vi "Halvorsen_HDiagram_BasicMethods.vi"(11 "Initial Conditions":ext[](array[numeric])=[0.1, 0.1, 0.1]) -> ()   [LabVIEW 2016]
panel:
  out "Current h":ext=0.9999999999999999994
  in  "Inc h, с":ext=0.01
  in  "Parameters":ext[](array[numeric])=[0.1, 0.0, 0.1]
  in  "Tab Control":enum32{"Mode Analysis", "Time Domain"}(tab)=enum."Time Domain"
  out "Mode Analysis":cluster{ext[], dbl[]}[](graph)=[{[0.01, 0.02, 0.03, 0.04, 0.049999999999999999997, 0.059999999999999999995, 0.069999999999999999993, 0.07999999999999999999, 0.08999999999999999999, 0.09999999999999999999, 0.109999999999999999986, 0.119999999999999999984, 0.12999999999999999998, 0.13999999999999999999, 0.14999999999999999999, 0.16, 0.17, 0.18000000000000000001, 0.19000000000000000001, 0.20000000000000000002, 0.21000000000000000002, 0.22000000000000000003, 0.23000000000000000003, 0.24000000000000000004, 0.25000000000000000003, 0.26000000000000000002, 0.27000000000000000001, 0.28, 0.29, 0.29999999999999999998, 0.30999999999999999998, 0.31999999999999999997, 0.32999999999999999996, 0.33999999999999999995, 0.34999999999999999994, 0.35999999999999999993, 0.36999999999999999992, 0.37999999999999999991, 0.3899999999999999999, 0.3999999999999999999, 0.40999999999999999989, 0.41999999999999999988, 0.42999999999999999987, 0.43999999999999999986, 0.44999999999999999985, 0.45999999999999999984, 0.46999999999999999984, 0.47999999999999999983, 0.48999999999999999982, 0.4999999999999999998, 0.50999999999999999983, 0.51999999999999999982, 0.5299999999999999998, 0.5399999999999999998, 0.5499999999999999998, 0.5599999999999999998, 0.56999999999999999978, 0.57999999999999999977, 0.58999999999999999976, 0.59999999999999999975, 0.60999999999999999974, 0.61999999999999999973, 0.62999999999999999972, 0.6399999999999999997, 0.6499999999999999997, 0.6599999999999999997, 0.6699999999999999997, 0.67999999999999999968, 0.68999999999999999967, 0.69999999999999999966, 0.70999999999999999966, 0.71999999999999999965, 0.72999999999999999964, 0.73999999999999999963, 0.74999999999999999962, 0.7599999999999999996, 0.7699999999999999996, 0.7799999999999999996, 0.7899999999999999996, 0.79999999999999999958, 0.80999999999999999957, 0.81999999999999999956, 0.82999999999999999955, 0.83999999999999999954, 0.84999999999999999953, 0.85999999999999999953, 0.8699999999999999995, 0.8799999999999999995, 0.8899999999999999995, 0.8999999999999999995, 0.9099999999999999995, 0.91999999999999999947, 0.92999999999999999946, 0.93999999999999999946, 0.94999999999999999945, 0.95999999999999999944, 0.96999999999999999943, 0.9799999999999999994, 0.9899999999999999994], [1.0, 1.0, 1.0, 1.0, 1.0, 1.0, 1.0, 1.0, 1.0, 1.0, 1.0, 1.0, 1.0, 1.0, 1.0, 1.0, 1.0, 1.0, 1.0, 1.0, 1.0, 1.0, 1.0, 1.0, 1.0, 1.0, 1.0, 1.0, 1.0, 1.0, 1.0, 1.0, 1.0, 1.0, 1.0, 1.0, 1.0, 1.0, 1.0, 1.0, 1.0, 1.0, 1.0, 1.0, 1.0, 1.0, 1.0, 1.0, 1.0, 1.0, 1.0, 1.0, 1.0, 1.0, 1.0, 1.0, 1.0, 1.0, 1.0, 1.0, 1.0, 1.0, 1.0, 1.0, 1.0, 1.0, 1.0, 1.0, 1.0, 1.0, 1.0, 22.0, 1.0, 1.0, 1.0, 1.0, 1.0, 18.0, 1.0, 1.0, 1.0, 1.0, 1.0, 1.0, 1.0, 1.0, 1.0, 24.0, 1.0, 1.0, 1.0, 1.0, 1.0, 1.0, 1.0, 1.0, 1.0, 1.0, 1.0]}, {[0.01, 0.02, 0.03, 0.04, 0.049999999999999999997, 0.059999999999999999995, 0.069999999999999999993, 0.07999999999999999999, 0.08999999999999999999, 0.09999999999999999999, 0.109999999999999999986, 0.119999999999999999984, 0.12999999999999999998, 0.13999999999999999999, 0.14999999999999999999, 0.16, 0.17, 0.18000000000000000001, 0.19000000000000000001, 0.20000000000000000002, 0.21000000000000000002, 0.22000000000000000003, 0.23000000000000000003, 0.24000000000000000004, 0.25000000000000000003, 0.26000000000000000002, 0.27000000000000000001, 0.28, 0.29, 0.29999999999999999998, 0.30999999999999999998, 0.31999999999999999997, 0.32999999999999999996, 0.33999999999999999995, 0.34999999999999999994, 0.35999999999999999993, 0.36999999999999999992, 0.37999999999999999991, 0.3899999999999999999, 0.3999999999999999999, 0.40999999999999999989, 0.41999999999999999988, 0.42999999999999999987, 0.43999999999999999986, 0.44999999999999999985, 0.45999999999999999984, 0.46999999999999999984, 0.47999999999999999983, 0.48999999999999999982, 0.4999999999999999998, 0.50999999999999999983, 0.51999999999999999982, 0.5299999999999999998, 0.5399999999999999998, 0.5499999999999999998, 0.5599999999999999998, 0.56999999999999999978, 0.57999999999999999977, 0.58999999999999999976, 0.59999999999999999975, 0.60999999999999999974, 0.61999999999999999973, 0.62999999999999999972, 0.6399999999999999997, 0.6499999999999999997, 0.6599999999999999997, 0.6699999999999999997, 0.67999999999999999968, 0.68999999999999999967, 0.69999999999999999966, 0.70999999999999999966, 0.71999999999999999965, 0.72999999999999999964, 0.73999999999999999963, 0.74999999999999999962, 0.7599999999999999996, 0.7699999999999999996, 0.7799999999999999996, 0.7899999999999999996, 0.79999999999999999958, 0.80999999999999999957, 0.81999999999999999956, 0.82999999999999999955, 0.83999999999999999954, 0.84999999999999999953, 0.85999999999999999953, 0.8699999999999999995, 0.8799999999999999995, 0.8899999999999999995, 0.8999999999999999995, 0.9099999999999999995, 0.91999999999999999947, 0.92999999999999999946, 0.93999999999999999946, 0.94999999999999999945, 0.95999999999999999944, 0.96999999999999999943, 0.9799999999999999994, 0.9899999999999999994], [0.0, 0.0, 0.0, 0.0, 0.0, 0.0, 0.0, 0.0, 0.0, 0.0, 0.0, 0.0, 0.0, 0.0, 0.0, 0.0, 0.0, 0.0, 0.0, 0.0, 0.0, 0.0, 0.0, 0.0, 0.0, 0.0, 0.0, 0.0, 0.0, 0.0, 0.0, 0.0, 0.0, 0.0, 0.0, 0.0, 0.0, 0.0, 0.0, 0.0, 0.0, 0.0, 0.0, 0.0, 0.0, 0.0, 0.0, 0.0, 0.0, 0.0, 0.0, 0.0, 0.0, 0.0, 0.0, 0.0, 0.0, 0.0, 0.0, 0.0, 0.0, 0.0, 0.0, 0.0, 0.0, 0.0, 0.0, 0.0, 0.0, 0.0, 0.0, 22.0, 0.0, 0.0, 0.0, 0.0, 0.0, 18.0, 0.0, 0.0, 0.0, 0.0, 0.0, 0.0, 0.0, 0.0, 0.0, 22.0, 0.0, 0.0, 0.0, 0.0, 0.0, 0.0, 0.0, 0.0, 0.0, 0.0, 0.0]}]
  out "Waveform Graph":ext[][](graph)
  out "Bifurcation Diagram":cluster{ext[], ext[]}(graph)={[0.71999999999999999965, 0.71999999999999999965, 0.71999999999999999965, 0.71999999999999999965, 0.71999999999999999965, 0.71999999999999999965, 0.71999999999999999965, 0.71999999999999999965, 0.71999999999999999965, 0.71999999999999999965, 0.71999999999999999965, 0.71999999999999999965, 0.71999999999999999965, 0.71999999999999999965, 0.71999999999999999965, 0.71999999999999999965, 0.71999999999999999965, 0.71999999999999999965, 0.71999999999999999965, 0.71999999999999999965, 0.71999999999999999965, 0.71999999999999999965, 0.71999999999999999965, 0.7799999999999999996, 0.7799999999999999996, 0.7799999999999999996, 0.7799999999999999996, 0.7799999999999999996, 0.7799999999999999996, 0.7799999999999999996, 0.7799999999999999996, 0.7799999999999999996, 0.7799999999999999996, 0.7799999999999999996, 0.7799999999999999996, 0.7799999999999999996, 0.7799999999999999996, 0.7799999999999999996, 0.7799999999999999996, 0.7799999999999999996, 0.7799999999999999996, 0.7799999999999999996, 0.7799999999999999996, 0.7799999999999999996, 0.8799999999999999995, 0.8799999999999999995, 0.8799999999999999995, 0.8799999999999999995, 0.8799999999999999995, 0.8799999999999999995, 0.8799999999999999995, 0.8799999999999999995, 0.8799999999999999995, 0.8799999999999999995, 0.8799999999999999995, 0.8799999999999999995, 0.8799999999999999995, 0.8799999999999999995, 0.8799999999999999995, 0.8799999999999999995, 0.8799999999999999995, 0.8799999999999999995, 0.8799999999999999995, 0.8799999999999999995, 0.8799999999999999995, 0.8799999999999999995, 0.8799999999999999995, 0.8799999999999999995, 0.8799999999999999995, 0.8799999999999999995, 0.8799999999999999995], [0.639111014809406, 4.833867372753233, 2.437827329373398, 5.464587799575122, 1.957741051925766, 4.511723895781915, 5.157315472089383, 5.0405567556074224, 5.188146836719836, 0.4062278567384584, 0.37024795742955646, 0.4987700730013437, 0.4269380981137045, 0.39272484974785477, 0.6072349133942436, 0.23944130553022655, 3.0099217859072844, 0.9956162659466771, 3.117694884263246, 1.1491520320780864, 7.575634158086566, 3.5490545539303584, 1.796520461112184, 3.1850454295908284, 0.13675466345870352, 4.024843393836113, 4.102728218253517, 0.6705460633442852, 4.763437644187874, 3.0400375849914845, 1.3900198763237597, 3.619218652213499, 5.716231022115606, 4.025224034358953, 4.22012460093736, 0.14242561841741205, 1.8182477129681602, 1.7115597064600077, 2.3566879769841598, 2.894364839995037, 2.6065703379241145, 1.2922508252315623, 4.678616310240351, 4.011654788354844, 2.2932165791100707, 5.639833400593374, 1.2366205946302218, 2.3574338767222764, 4.256024403109746, 4.633942953034731, 2.9958747226369784, 1.512375597751331, 2.9432515471835465, 0.8994817871400373, 0.6295734696668136, 4.743878365327232, 3.241155630915066, 2.0290566391301805, 2.3049992005414466, 2.9243987652286645, 3.0777550328644123, 0.20526761969285426, 3.9525478928381053, 1.9100921915966034, 1.7025794775643877, 2.321048458169814, 2.905257945224514, 2.8336287848779524, 3.0797848283852893, 0.21402653087164758, 3.963566483752086]}
  in  "Final h":dbl=1.0
  in  "Variable":u16(ring) items=["x", "y", "z"]
  in  "Время, с":ext=500.0
  in  "Шаг h, с":ext=0.01
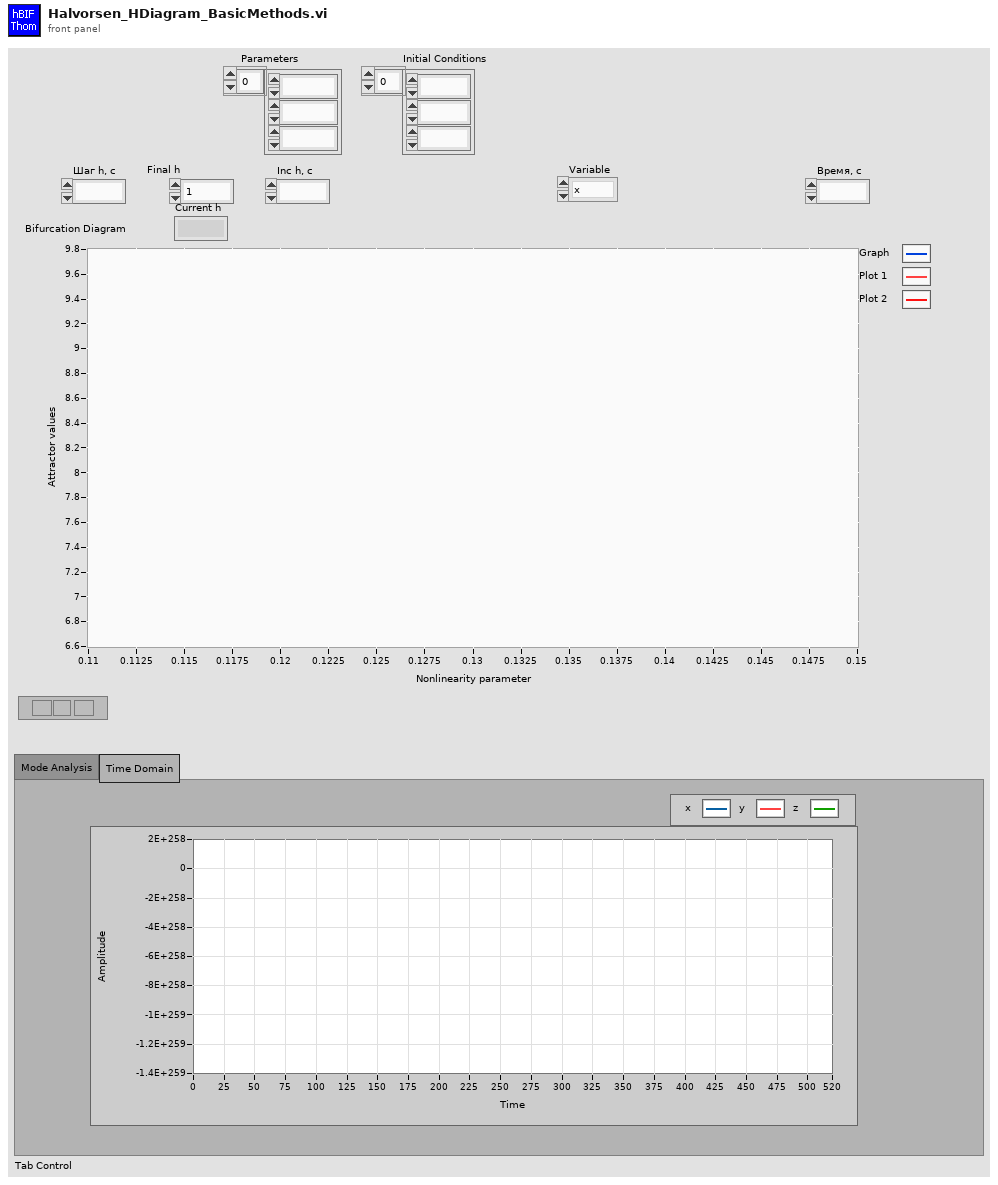
[diagram p1: front panel]
types:
  T1 = enum16{"Euler", "Cromer 1", "Cromer 2", "D1", "D2", "PD1", "PD2", "CD1", "CD2", "CD3", "CD4", "IMP", "LIMP", "IEuler", "SEMP", "SIMP", "EMP", "MEMP"}
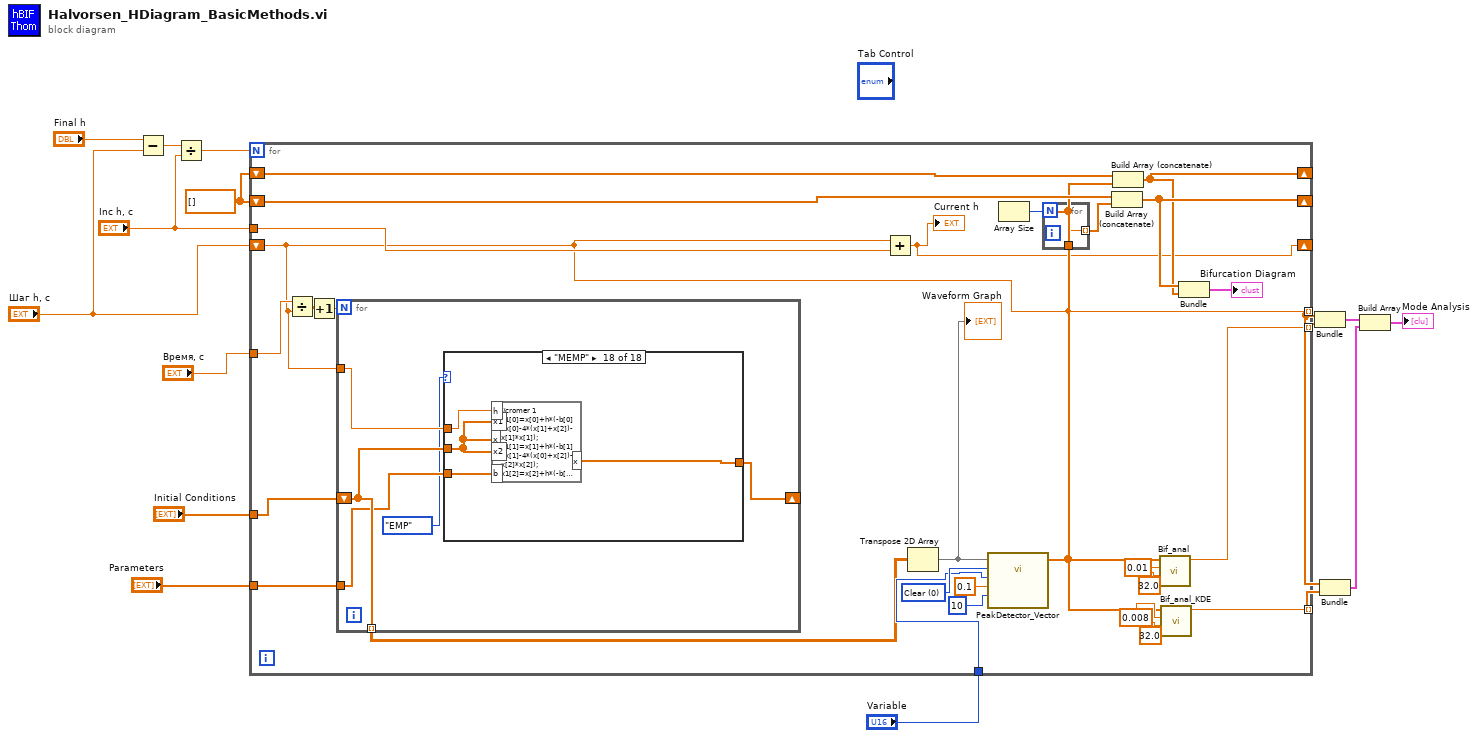
[diagram p0: block diagram]
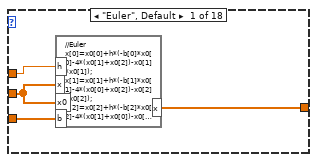
[diagram p2: hidden frame]
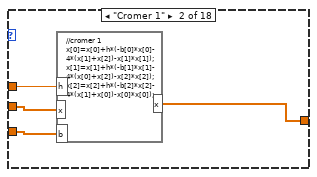
[diagram p3: hidden frame]
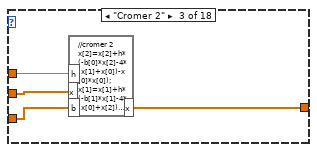
[diagram p4: hidden frame]
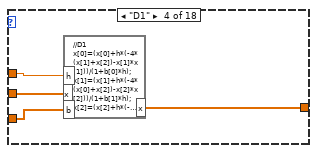
[diagram p5: hidden frame]
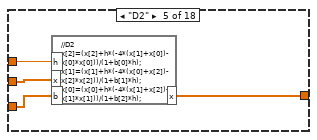
[diagram p6: hidden frame]
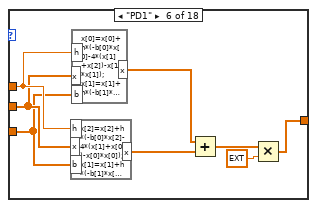
[diagram p7: hidden frame]
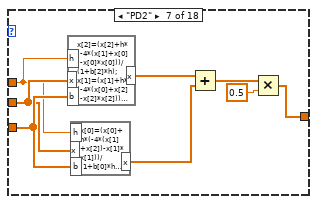
[diagram p8: hidden frame]
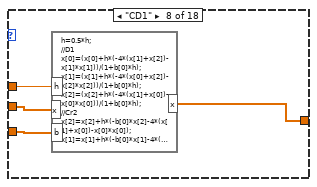
[diagram p9: hidden frame]
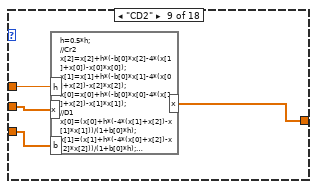
[diagram p10: hidden frame]
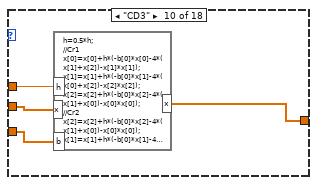
[diagram p11: hidden frame]
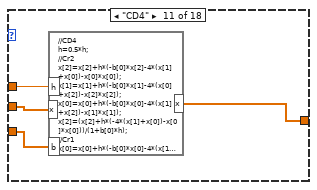
[diagram p12: hidden frame]
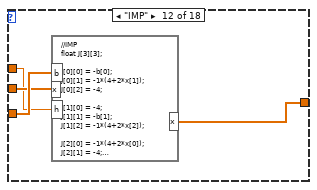
[diagram p13: hidden frame]
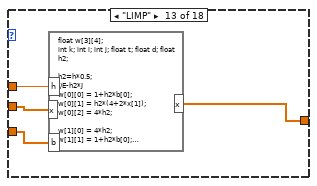
[diagram p14: hidden frame]
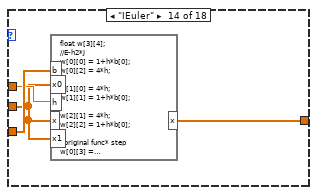
[diagram p15: hidden frame]
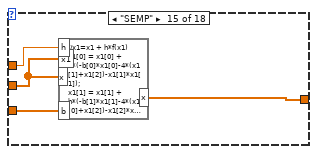
[diagram p16: hidden frame]
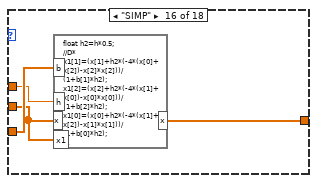
[diagram p17: hidden frame]
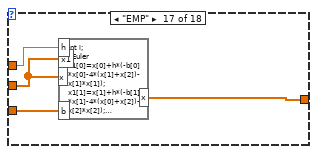
[diagram p18: hidden frame]
diagram:
  w13 = ext[] []
  n1 = Subtract(x="Final h", y="Шаг h, с") -> (x-y=w4:ext)
  n2 = Divide(x=w4, y="Inc h, с") -> (x/y=w2:ext)
  n3 = for {
    N: w2 -> [_]
    tunnel: "Время, с" -> [w21]
    tunnel: "Initial Conditions" -> [w23]
    shift-right: [w24] -> _
    shift-left: "Шаг h, с" -> [w17]
    tunnel: [w41] -> w12 mode=indexing
    tunnel: "Variable" -> [w40]
    shift-right: [w33] -> _
    shift-left: w13 -> [w38]
    shift-right: [w34] -> _
    shift-left: w13 -> [w37]
    tunnel: [w17] -> w9 mode=indexing
    tunnel: [w27] -> w8 mode=indexing
    tunnel: "Parameters" -> [w22]
    tunnel: "Inc h, с" -> [w25]
    w44 = u16 0 items=["Clear", "Absolute", "Positive"] ("Signal Mode")
    n4 = Divide(x=w21, y=w17) -> (x/y=w19:ext)
    n5 = Increment(x=w19) -> (x+1=w18:ext)
    n6 = for {
      N: w18 -> [_]
      shift-right: [w45] -> _
      shift-left: w23 -> [w48]
      tunnel: w22 -> [w47]
      tunnel: w17 -> [w49]
      tunnel: [w48] -> w20 mode=indexing
      n7 = case shown="\"MEMP\"" T1."EMP" ("Method") {
        tunnel: w49 -> [w51 w57 w60 w64 w69 w72 w78 w88 w92 w97 w100 w102 w109 w112 w116 w119 w123 w127]
        tunnel: w47 -> [w53 w55 w58 w62 w67 w70 w80 w86 w90 w95 w98 w104 w106 w113 w114 w120 w124 w128]
        tunnel: w48 -> [w52 w56 w59 w63 w68 w71 w79 w87 w91 w96 w99 w103 w107 w111 w115 w118 w122 w129]
        tunnel: [w50 w54 w61 w65 w66 w73 w81 w89 w93 w94 w101 w105 w108 w110 w117 w121 w125 w126] -> w45
        frame "Euler", Default {
          n8 = formula code="//Euler\nx[0]=x0[0]+h*(-b[0]*x0[0]-4*(x0[1]+x0[2])-x0[1]*x0[1]);\nx[1]=x0[1]+h*(-b[1]*x0[1]-4*(x0[0]+x0[2])-x0[2]*x0[2]);\nx[2]=x0[2]+h*(-b[2]*x0[2]-4*(x0[1]+x0[0])-x0[0]*x0[0]);"("x"=w52, "x0"=w52, "b"=w53, "h"=w51) -> ("x"=w50:ext[])
        }
        frame "Cromer 1" {
          n9 = formula code="//cromer 1\nx[0]=x[0]+h*(-b[0]*x[0]-4*(x[1]+x[2])-x[1]*x[1]);\nx[1]=x[1]+h*(-b[1]*x[1]-4*(x[0]+x[2])-x[2]*x[2]);\nx[2]=x[2]+h*(-b[2]*x[2]-4*(x[1]+x[0])-x[0]*x[0]);"("x"=w56, "b"=w55, "h"=w57) -> ("x"=w54:ext[])
        }
        frame "Cromer 2" {
          n10 = formula code="//cromer 2\nx[2]=x[2]+h*(-b[0]*x[2]-4*(x[1]+x[0])-x[0]*x[0]);\nx[1]=x[1]+h*(-b[1]*x[1]-4*(x[0]+x[2])-x[2]*x[2]);\nx[0]=x[0]+h*(-b[2]*x[0]-4*(x[1]+x[2])-x[1]*x[1]);"("x"=w59, "b"=w58, "h"=w60) -> ("x"=w61:ext[])
        }
        frame "D1" {
          n11 = formula code="//D1\nx[0]=(x[0]+h*(-4*(x[1]+x[2])-x[1]*x[1]))/(1+b[0]*h);\nx[1]=(x[1]+h*(-4*(x[0]+x[2])-x[2]*x[2]))/(1+b[1]*h);\nx[2]=(x[2]+h*(-4*(x[1]+x[0])-x[0]*x[0]))/(1+b[2]*h);"("x"=w63, "b"=w62, "h"=w64) -> ("x"=w65:ext[])
        }
        frame "D2" {
          n12 = formula code="//D2\nx[2]=(x[2]+h*(-4*(x[1]+x[0])-x[0]*x[0]))/(1+b[0]*h);\nx[1]=(x[1]+h*(-4*(x[0]+x[2])-x[2]*x[2]))/(1+b[1]*h);\nx[0]=(x[0]+h*(-4*(x[1]+x[2])-x[1]*x[1]))/(1+b[2]*h);"("x"=w68, "b"=w67, "h"=w69) -> ("x"=w66:ext[])
        }
        frame "PD1" {
          n13 = formula code="x[2]=x[2]+h*(-b[0]*x[2]-4*(x[1]+x[0])-x[0]*x[0]);\nx[1]=x[1]+h*(-b[1]*x[1]-4*(x[0]+x[2])-x[2]*x[2]);\nx[0]=x[0]+h*(-b[2]*x[0]-4*(x[1]+x[2])-x[1]*x[1]);"("x"=w71, "b"=w70, "h"=w72) -> ("x"=w75:ext[])
          n14 = formula code="x[0]=x[0]+h*(-b[0]*x[0]-4*(x[1]+x[2])-x[1]*x[1]);\nx[1]=x[1]+h*(-b[1]*x[1]-4*(x[0]+x[2])-x[2]*x[2]);\nx[2]=x[2]+h*(-b[2]*x[2]-4*(x[1]+x[0])-x[0]*x[0]);"("x"=w71, "b"=w70, "h"=w72) -> ("x"=w74:ext[])
          n15 = Add(x=w74, y=w75) -> (x+y=w76:ext[])
          n16 = Multiply(x=w76, y=ext 0.5) -> (x*y=w73:ext[])
        }
        frame "PD2" {
          n17 = formula code="x[2]=(x[2]+h*(-4*(x[1]+x[0])-x[0]*x[0]))/(1+b[2]*h);\nx[1]=(x[1]+h*(-4*(x[0]+x[2])-x[2]*x[2]))/(1+b[1]*h);\nx[0]=(x[0]+h*(-4*(x[1]+x[2])-x[1]*x[1]))/(1+b[0]*h);"("x"=w79, "b"=w80, "h"=w78) -> ("x"=w85:ext[])
          n18 = formula code="x[0]=(x[0]+h*(-4*(x[1]+x[2])-x[1]*x[1]))/(1+b[0]*h);\nx[1]=(x[1]+h*(-4*(x[0]+x[2])-x[2]*x[2]))/(1+b[0]*h);\nx[2]=(x[2]+h*(-4*(x[1]+x[0])-x[0]*x[0]))/(1+b[0]*h);"("x"=w79, "b"=w80, "h"=w78) -> ("x"=w84:ext[])
          n19 = Add(x=w85, y=w84) -> (x+y=w83:ext[])
          n20 = Multiply(x=w83, y=0.5) -> (x*y=w81:ext[])
        }
        frame "CD1" {
          n21 = formula code="h=0.5*h;\n//D1\nx[0]=(x[0]+h*(-4*(x[1]+x[2])-x[1]*x[1]))/(1+b[0]*h);\nx[1]=(x[1]+h*(-4*(x[0]+x[2])-x[2]*x[2]))/(1+b[0]*h);\nx[2]=(x[2]+h*(-4*(x[1]+x[0])-x[0]*x[0]))/(1+b[0]*h);\n//Cr2\nx[2]=x[2]+h*(-b[0]*x[2]-4*(x[1]+x[0])-x[0]*x[0]);\nx[1]=x[1]+h*(-b[0]*x[1]-4*(x[0]+x[2])-x[2]*x[2]);\nx[0]=x[0]+h*(-b[0]*x[0]-4*(x[1]+x[2])-x[1]*x[1]);"("x"=w87, "b"=w86, "h"=w88) -> ("x"=w89:ext[])
        }
        frame "CD2" {
          n22 = formula code="h=0.5*h;\n//Cr2\nx[2]=x[2]+h*(-b[0]*x[2]-4*(x[1]+x[0])-x[0]*x[0]);\nx[1]=x[1]+h*(-b[0]*x[1]-4*(x[0]+x[2])-x[2]*x[2]);\nx[0]=x[0]+h*(-b[0]*x[0]-4*(x[1]+x[2])-x[1]*x[1]);\n//D1\nx[0]=(x[0]+h*(-4*(x[1]+x[2])-x[1]*x[1]))/(1+b[0]*h);\nx[1]=(x[1]+h*(-4*(x[0]+x[2])-x[2]*x[2]))/(1+b[0]*h);\nx[2]=(x[2]+h*(-4*(x[1]+x[0])-x[0]*x[0]))/(1+b[0]*h);"("x"=w91, "b"=w90, "h"=w92) -> ("x"=w93:ext[])
        }
        frame "CD3" {
          n23 = formula code="h=0.5*h;\n//Cr1\nx[0]=x[0]+h*(-b[0]*x[0]-4*(x[1]+x[2])-x[1]*x[1]);\nx[1]=x[1]+h*(-b[0]*x[1]-4*(x[0]+x[2])-x[2]*x[2]);\nx[2]=x[2]+h*(-b[0]*x[2]-4*(x[1]+x[0])-x[0]*x[0]);\n//Cr2\nx[2]=x[2]+h*(-b[0]*x[2]-4*(x[1]+x[0])-x[0]*x[0]);\nx[1]=x[1]+h*(-b[0]*x[1]-4*(x[0]+x[2])-x[2]*x[2]);\nx[0]=x[0]+h*(-b[0]*x[0]-4*(x[1]+x[2])-x[1]*x[1]);"("x"=w96, "b"=w95, "h"=w97) -> ("x"=w94:ext[])
        }
        frame "CD4" {
          n24 = formula code="//CD4\nh=0.5*h;\n//Cr2\nx[2]=x[2]+h*(-b[0]*x[2]-4*(x[1]+x[0])-x[0]*x[0]);\nx[1]=x[1]+h*(-b[0]*x[1]-4*(x[0]+x[2])-x[2]*x[2]);\nx[0]=x[0]+h*(-b[0]*x[0]-4*(x[1]+x[2])-x[1]*x[1]);\nx[2]=(x[2]+h*(-4*(x[1]+x[0])-x[0]*x[0]))/(1+b[0]*h);\n//Cr1\nx[0]=x[0]+h*(-b[0]*x[0]-4*(x[1]+x[2])-x[1]*x[1]);\nx[1]=x[1]+h*(-b[0]*x[1]-4*(x[0]+x[2])-x[2]*x[2]);\nx[2]=x[2]+h*(-b[0]*x[2]-4*(x[1]+x[0])-x[0]*x[0]);"("x"=w99, "b"=w98, "h"=w100) -> ("x"=w101:ext[])
        }
        frame "IMP" {
          n25 = formula code="//IMP\nfloat J[3][3];\n\nJ[0][0] = -b[0]; \nJ[0][1] = -1*(4+2*x[1]); \nJ[0][2] = -4; \n\nJ[1][0] = -4; \nJ[1][1] = -b[1];\nJ[1][2] = -1*(4+2*x[2]);\n\nJ[2][0] = -1*(4+2*x[0]); \nJ[2][1] = -4;\nJ[2][2] = -b[2];\n\n\nfloat w[3][4], Z[3], a[3], Zn[3], dz;\nfloat tol;\nint k; int i; int j; float t; float d;\ntol = 1e-14;\nint nnewtmax = 3, nnewt;\ndz = 2e-13;\nnnewt = 0;\n\nZ[0] = x[0]; Z[1] = x[1]; Z[2] = x[2];\nwhile ( (dz > tol) && (nnewt < nnewtmax)){\n\tfor(i=0;i<3;i++)\n\t{\n\t\tfor(j=0;j<3;j++)\n\t\t{\n\t\t\tif (i==j)\n\t\t\tw[i][j]=1 - 0.5*h*J[i][j];\n\t\t\telse\n\t\t\tw[i][j]= - 0.5*h*J[i][j];\n\t\t}\n\t}\n\n\n\n\ta[0] = 0.5*(x[0] + Z[0]);\n\ta[1] = 0.5*(x[1] + Z[1]);\n\ta[2] = 0.5*(x[2] + Z[2]);\n\t\n\tw[0][3]= -Z[0]+x[0]+h*(-b[0]*a[0]-4*(a[1]+a[2])-a[1]*a[1]);\n\tw[1][3]= -Z[1]+x[1]+h*(-b[1]*a[1]-4*(a[0]+a[2])-a[2]*a[2]);\n\tw[2][3]= -Z[2]+x[2]+h*(-b[2]*a[2]-4*(a[1]+a[0])-a[0]*a[0]);\n\t\n\t\n\tfor(k = 0; k <= 1; k++){\n\t\tint l = k;\n\t\n\t\tfor( i = k+1; i<= 2; i++){\n\t\t\tif( abs(w[i][k]) > abs(w[l][k]) ){\n\t\t\tl = i;\n\t\t\t}\n\t\t}\n\t\tif (l != k){\n\t\t\tfor( j = 0; j <= 3; j++){\n\t\t\t\tif ((j == 0) || (j >= k)){\n\t\t\t\t\tt = w[k][j];\n\t\t\t\t\tw[k][j] = w[l][j];\n\t\t\t\t\tw[l][j] = t;\n\t\t\t\t}\n\t\t\t}\n\t\t}\t\n\n\t\td = 1.0 / w[k][k];\n\t\tfor( i=(k+1); i <=(2); i++){\n\t\t\tif (w[i][k] == 0){\n\t\t\t\tcontinue;\n\t\t\t}\n\t\t\tt = w[i][k] * d;\n\t\t\tfor ( j = k; j <= (3); j++) {\n\t\t\t\tif (w[k][j] != 0){\n\t\t\t\t\tw[i][j] = w[i][j] - t * w[k][j];\n\t\t\t\t}\n\t\t\t}\n\t\t}\n\t}\n\tfor( i=(3); i >= 2; i--){\n\t\tfor( j=1; j <= i-1; j++){\n\t\t\tt = w[i - j - 1][i - 1]/w[ i -1][i - 1];\n\t\t\tw[i-j - 1][ 3] = w[i-j -1][3] - t*w[i - 1][ 3];\n\t\t}\n\t\tw[i-1][ 3] = w[i - 1][3]/w[ i -1][i - 1];\n\t}\n\tw[0][3] = w[0][3]/w[0][0];\n\tZn[0] = Z[0]+ w[0][3];\n\tZn[1] = Z[1]+ w[1][3];\n\tZn[2] = Z[2]+ w[2][3];\n\t\n\tdz = ( (Zn[0] - Z[0])**2 + (Zn[1] - Z[1])**2 + (Zn[2] - Z[2])**2 )**0.5;\n\tZ[0] = Zn[0];\n\tZ[1] = Zn[1];\n\tZ[2] = Zn[2];\n\n\tnnewt ++;\n}\n\nx[0] = Zn[0];\nx[1] = Zn[1];\nx[2] = Zn[2];"("x"=w103, "h"=w102, "b"=w104) -> ("x"=w105:ext[])
        }
        frame "LIMP" {
          n26 = formula code="float w[3][4];\nint k; int i; int j; float t; float d; float h2;\n\nh2=h*0.5;\n//E-h2*J\nw[0][0] = 1+h2*b[0];\nw[0][1] = h2*(4+2*x[1]);\nw[0][2] = 4*h2;\n\nw[1][0] = 4*h2;\nw[1][1] = 1+h2*b[0];\nw[1][2] = h2*(4+2*x[2]);\n\nw[2][0] = h2*(4+2*x[0]);\nw[2][1] = 4*h2;\nw[2][2] = 1+h2*b[0];\n\n//original func* step\nw[0][3] = h*(-b[0]*x[0]-4*(x[1]+x[2])-x[1]*x[1]);\nw[1][3] = h*(-b[0]*x[1]-4*(x[0]+x[2])-x[2]*x[2]);\nw[2][3] = h*(-b[0]*x[2]-4*(x[1]+x[0])-x[0]*x[0]);\n\n\nint HEIGHT = 3;\nint  WIDTH = 4;\nfor(k = 0; k <= HEIGHT-2; k++){\n\nint\tl = k;\n\nfor( i = k+1;  i<= HEIGHT-1; i++){\n\t\t\tif( abs(w[i][k]) > abs(w[l][k]) ){\n\t\t\t\tl = i;\n    }\n   }\n\t\tif (l != k){\n\t\t\tfor( j = 0; j <= WIDTH-1; j++){\n\t\t\t\tif ((j == 0) || (j >= k)){\n\t\t\t\t\tt = w[k][j];\n\t\t\t\t\tw[k][j] = w[l][j];\n\t\t\t\t\tw[l][j] = t;\n                }\n            }\n        }\n\n\t\td = 1.0 / w[k][k];\n\t\tfor( i=(k+1); i <=(HEIGHT-1); i++){\n\t\t\tif (w[i][k] == 0){\n                continue;\n            }\n\t\t\tt = w[i][k] * d;\n\t\t\tfor ( j = k; j <= (WIDTH-1); j++) {\n\t\t\t\tif (w[k][j] != 0){\n\t\t\t\t\tw[i][j] = w[i][j] - t * w[k][j];\n                }\n            }\n        }\n    }\n    \n\t\n    for( i=(HEIGHT); i >= 2; i--){ \n        for( j=1; j <= i-1; j++){\n            t = w[i - j - 1][i - 1]/w[ i -1][i - 1];\n            w[i-j - 1][ WIDTH- 1] = w[i-j -1][ WIDTH -1] - t*w[i - 1][ WIDTH -1];\n        }\n        w[i-1][ WIDTH-1] = w[i - 1][ WIDTH - 1]/w[ i -1][i - 1];\n    }\n    w[0][ WIDTH - 1] = w[0][ WIDTH -1]/w[0][0];\n\n    \n    x[0] =x[0]+ w[0][WIDTH - 1];\n    x[1] = x[1]+w[1][WIDTH - 1];\n    x[2] = x[2]+w[2][WIDTH - 1];"("x"=w107, "b"=w106, "h"=w109) -> ("x"=w108:ext[])
        }
        frame "IEuler" {
          n27 = formula code="float w[3][4];\n//E-h2*J\nw[0][0] = 1+h*b[0];\nw[0][2] = 4*h;\n\nw[1][0] = 4*h;\nw[1][1] = 1+h*b[0];\n\nw[2][1] = 4*h;\nw[2][2] = 1+h*b[0];\n\n//original func* step\nw[0][3] = h*(-b[0]*x[0]-4*(x[1]+x[2])-x[1]*x[1]);\nw[1][3] = h*(-b[0]*x[1]-4*(x[0]+x[2])-x[2]*x[2]);\nw[2][3] = h*(-b[0]*x[2]-4*(x[1]+x[0])-x[0]*x[0]);\n\nfloat tol = 1e-12;\nfloat dx = 2*tol;\n\nint nmax = 10;\nint n = 0;\n//цикл по Ньютонам\nwhile ((dx > tol)&&(n < nmax)){\n\n\tw[0][1] = h*(4+2*x[1]);\n\tw[1][2] = h*(4+2*x[2]);\n\tw[2][0] = h*(4+2*x[0]);\n\n\tw[0][3] = x0[0] - x1[0] + h*(-b[0]*x[0]-4*(x[1]+x[2])-x[1]*x[1]);\n\tw[1][3] = x0[1] - x1[1] + h*(-b[0]*x[1]-4*(x[0]+x[2])-x[2]*x[2]);\n\tw[2][3] = x0[2] - x1[2] + h*(-b[0]*x[2]-4*(x[1]+x[0])-x[0]*x[0]);\n\n\tint HEIGHT = 3;\n\tint  WIDTH = 4;\n\tint k; int i; int j; float t; float d;\n\n\tfor(k = 0; k <= HEIGHT-2; k++){\n\t\tint\tl = k;\n\t\tfor( i = k+1;  i<= HEIGHT-1; i++){\n\t\t\t\t\tif( abs(w[i][k]) > abs(w[l][k]) ){\n\t\t\t\t\t\tl = i;\n\t\t\t}\n\t   }\n\t\t\tif (l != k){\n\t\t\t\tfor( j = 0; j <= WIDTH-1; j++){\n\t\t\t\t\tif ((j == 0) || (j >= k)){\n\t\t\t\t\t\tt = w[k][j];\n\t\t\t\t\t\tw[k][j] = w[l][j];\n\t\t\t\t\t\tw[l][j] = t;\n\t\t\t\t\t}\n\t\t\t\t}\n\t\t\t}\n\t\t\t\n\t\t\td = 1.0 / w[k][k];\n\t\t\tfor( i=(k+1); i <=(HEIGHT-1); i++){\n\t\t\t\tif (w[i][k] == 0){\n\t\t\t\t\tcontinue;\n\t\t\t\t}\n\t\t\t\tt = w[i][k] * d;\n\t\t\t\tfor ( j = k; j <= (WIDTH-1); j++) {\n\t\t\t\t\tif (w[k][j] != 0){\n\t\t\t\t\t\tw[i][j] = w[i][j] - t * w[k][j];\n\t\t\t\t\t}\n\t\t\t\t}\n\t\t\t}\n\t\t}\n\n\t\tfor( i=(HEIGHT); i >= 2; i--){ \n\t\t\tfor( j=1; j <= i-1; j++){\n\t\t\t\tt = w[i - j - 1][i - 1]/w[ i -1][i - 1];\n\t\t\t\tw[i-j - 1][ WIDTH- 1] = w[i-j -1][ WIDTH -1] - t*w[i - 1][ WIDTH -1];\n\t\t\t}\n\t\t\tw[i-1][ WIDTH-1] = w[i - 1][ WIDTH - 1]/w[ i -1][i - 1];\n\t\t}\n\t\tw[0][ WIDTH - 1] = w[0][ WIDTH -1]/w[0][0];\n\n\t\t\n\t\tx1[0] =x[0]+ w[0][WIDTH - 1];\n\t\tx1[1] = x[1]+w[1][WIDTH - 1];\n\t\tx1[2] = x[2]+w[2][WIDTH - 1];\n\n\tdx = sqrt((x1[0] - x[0])**2 + (x1[1] - x[1])**2 + (x1[2] - x[2])**2);\n\tn++;\n\n\tx[0] = x1[0]; x[1] = x1[1]; x[2] = x1[2];\n\n}"("x"=w111, "h"=w112, "x1"=w111, "b"=w113, "x0"=w111) -> ("x"=w110:ext[])
        }
        frame "SEMP" {
          n28 = formula code="//x1=x1 + h*f(x1)\nx1[0] = x1[0] + h*(-b[0]*x1[0]-4*(x1[1]+x1[2])-x1[1]*x1[1]); \nx1[1] = x1[1] + h*(-b[1]*x1[1]-4*(x1[0]+x1[2])-x1[2]*x1[2]); \nx1[2] = x1[2] + h*(-b[2]*x1[2]-4*(x1[1]+x1[0])-x1[0]*x1[0]);\n\n\n//x+h*f(x1)\nx[0] = x[0] + h*(-b[0]*x1[0]-4*(x1[1]+x1[2])-x1[1]*x1[1]); \nx[1] = x[1] + h*(-b[1]*x1[1]-4*(x1[0]+x1[2])-x1[2]*x1[2]); \nx[2] = x[2] + h*(-b[2]*x1[2]-4*(x1[1]+x1[0])-x1[0]*x1[0]);"("x"=w115, "x1"=w115, "h"=w116, "b"=w114) -> ("x"=w117:ext[])
        }
        frame "SIMP" {
          n29 = formula code="float h2=h*0.5;\n//D*\nx1[1]=(x[1]+h2*(-4*(x[0]+x[2])-x[2]*x[2]))/(1+b[1]*h2);\nx1[2]=(x[2]+h2*(-4*(x[1]+x[0])-x[0]*x[0]))/(1+b[2]*h2);\nx1[0]=(x[0]+h2*(-4*(x[1]+x[2])-x[1]*x[1]))/(1+b[0]*h2);\n\n\n//??\nx[0]=x[0]+h*(-b[0]*x1[0]-4*(x1[1]+x1[2])-x1[1]*x1[1]);\nx[1]=x[1]+h*(-b[1]*x1[1]-4*(x1[0]+x1[2])-x1[2]*x1[2]);\nx[2]=x[2]+h*(-b[2]*x1[2]-4*(x1[1]+x1[0])-x1[0]*x1[0]);"("x"=w118, "h"=w119, "x1"=w118, "b"=w120) -> ("x"=w121:ext[])
        }
        frame "EMP" {
          n30 = formula code="int i;\n//Euler\nx1[0]=x[0]+h*(-b[0]*x[0]-4*(x[1]+x[2])-x[1]*x[1]);\nx1[1]=x[1]+h*(-b[1]*x[1]-4*(x[0]+x[2])-x[2]*x[2]);\nx1[2]=x[2]+h*(-b[2]*x[2]-4*(x[1]+x[0])-x[0]*x[0]);\n\n//EEuler\nx[0]=x[0]+h*(-b[0]*x1[0]-4*(x1[1]+x1[2])-x1[1]*x1[1]);\nx[1]=x[1]+h*(-b[1]*x1[1]-4*(x1[0]+x1[2])-x1[2]*x1[2]);\nx[2]=x[2]+h*(-b[2]*x1[2]-4*(x1[1]+x1[0])-x1[0]*x1[0]);"("x"=w122, "x1"=w122, "h"=w123, "b"=w124) -> ("x"=w125:ext[])
        }
        frame "MEMP" {
          n31 = formula code="//cromer 1\nx1[0]=x[0]+h*(-b[0]*x[0]-4*(x[1]+x[2])-x[1]*x[1]);\nx1[1]=x[1]+h*(-b[1]*x[1]-4*(x[0]+x[2])-x[2]*x[2]);\nx1[2]=x[2]+h*(-b[2]*x[2]-4*(x[1]+x[0])-x[0]*x[0]);\nh=2*h;\n\n//EEuler\nx2[0]=x[0]+h*(-b[0]*x1[0]-4*(x1[1]+x1[2])-x1[1]*x1[1]);\nx2[1]=x[1]+h*(-b[1]*x1[1]-4*(x1[0]+x1[2])-x1[2]*x1[2]);\nx2[2]=x[2]+h*(-b[2]*x1[2]-4*(x1[1]+x1[0])-x1[0]*x1[0]);\n\nx[0]=x1[0];\nx[1]=x1[1];\nx[2]=x1[2];\nx1[0]=x2[0];\nx1[1]=x2[1];\nx1[2]=x2[2];\nh=h*0.5;\nx[0]=(x[0]+x1[0]+h*(-b[0]*x1[0]-4*(x1[1]+x1[2])-x1[1]*x1[1]))/2;\nx[1]=(x[1]+x1[1]+h*(-b[1]*x1[1]-4*(x1[0]+x1[2])-x1[2]*x1[2]))/2;\nx[2]=(x[2]+x1[2]+h*(-b[2]*x1[2]-4*(x1[1]+x1[0])-x1[0]*x1[0]))/2;"("x"=w129, "x1"=w129, "h"=w127, "b"=w128, "x2"=w129) -> ("x"=w126:ext[])
        }
      }
    }
    n32 = Add(x=w17, y=w25) -> (x+y=w24:ext)
    "Current h" <- w24
    n33 = Transpose 2D Array(2D array=w20) -> (transposed array=w26:ext[][])
    "Waveform Graph" <- w26
    n34 = call "PeakDetector_Vector.vi"("threshold"=0.1, "FWD cut length"=10, "Variable_Num"=w40, "Signal Mode"=w44, "Input signal"=w26) -> ("Out signal"=w28:dbl[])  [unwired: 5 in, 1 out]
    n35 = Array Size(array=w28) -> (size(s)=w39:i32)
    n36 = for {
      N: w39 -> [_]
      tunnel: [w130] -> w35 mode=indexing
      tunnel: w17 -> [w130]
    }
    n37 = Build Array (concatenate)(w37, w35) -> (w34:ext[])
    n38 = Build Array (concatenate)(w38, w28) -> (w33:ext[])
    n39 = call "Bif_anal.vi"("n"=32.0, "Treshold"=0.01, "X"=w28) -> ("Y"=w41:dbl)  [unwired: 7 in, 1 out]
    n40 = call "Bif_anal_KDE.vi"("n"=32.0, "Manual h"=0.008 ("Treshold"), "X"=w28) -> ("Y"=w27:dbl)  [unwired: 7 in, 1 out]
    n41 = Bundle(w34, w33) -> (→"Bifurcation Diagram":cluster{ext[], ext[]})  [unwired: 1 in]
  }
  n42 = Bundle(w9, w12) -> (w11:cluster{ext[], dbl[]})  [unwired: 1 in]
  n43 = Bundle(w9, w8) -> (w7:cluster{ext[], dbl[]})  [unwired: 1 in]
  n44 = Build Array(w11, w7) -> (→"Mode Analysis":cluster{ext[], dbl[]}[])
